vi "tutorial-062_FromDLAY.vi"(11 "Control Array":refnum<vi>[](array[refnum])) -> ()   [LabVIEW 2019]
uses:
  TextControlledInstrum/TextControlledInstrum.lvlib
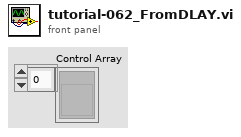
[diagram p1: front panel]
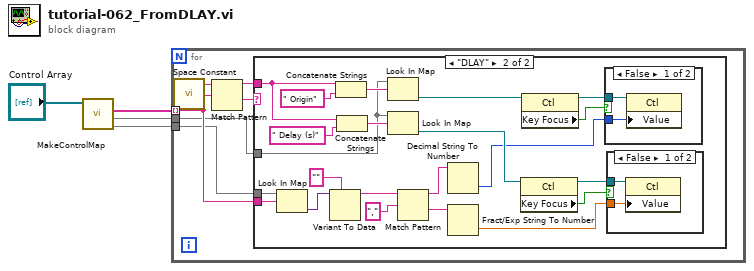
[diagram p0: block diagram]
diagram:
  n1 = call "MakeControlMap.vi"("ControlArray"="Control Array") -> ("ValueMap out"=w2:map{string, variant}, "ControlMap out"=w1:map{string, refnum<vi>}, "Names"=w3:string[])  [unwired: 7 in, 1 out]
  n2 = for {
    tunnel: w3 -> [w7] mode=indexing
    tunnel: w2 -> [w6]
    tunnel: w1 -> [w5]
    n3 = call <vilib>:"Space Constant.vi"() -> ("String"=w10:string)
    n4 = Match Pattern(string=w7, regular expression=w10) -> (before substring=w8:string, after substring=w9:string)  [unwired: 1 in, 2 out]
    n5 = case shown="\"DLAY\"" w9 {
      tunnel: w8 -> [_ w24]
      tunnel: w7 -> [_ w32]
      tunnel: w6 -> [_ w31]
      tunnel: w5 -> [_ w19]
      frame Default {
      }
      frame "DLAY" {
        n6 = Look In Map(map=w31, key=w32) -> (value=w25:variant)  [unwired: 1 in, 1 out]
        n7 = Variant To Data(type="", Variant=w25) -> (data=w26:string)  [unwired: 1 in, 1 out]
        n8 = Concatenate Strings(w24, " Origin") -> (w21:string)
        n9 = Concatenate Strings(w24, " Delay (s)") -> (w20:string)
        n10 = Look In Map(map=w19, key=w21) -> (value=w18:refnum<vi>)  [unwired: 1 in, 1 out]
        n11 = Look In Map(map=w19, key=w20) -> (value=w17:refnum<vi>)  [unwired: 1 in, 1 out]
        n12 = Match Pattern(string=w26, regular expression=",") -> (before substring=w27:string, after substring=w28:string)  [unwired: 1 in, 2 out]
        n13 = Decimal String To Number(string=w27) -> (number=w13:i32)  [unwired: 2 in, 1 out]
        n14 = Fract/Exp String To Number(string=w28) -> (number=w16:dbl)  [unwired: 3 in, 1 out]
        n15 = property class="Ctl"(reference=w17) -> (reference out=w14:refnum<vi>, "Key Focus"=w11:bool)  [unwired: 1 in, 1 out]
        n16 = property class="Ctl"(reference=w18) -> (reference out=w15:refnum<vi>, "Key Focus"=w12:bool)  [unwired: 1 in, 1 out]
        n17 = case shown="False" w12 {
          tunnel: w15 -> [w36 _]
          tunnel: w13 -> [w35 _]
          frame False {
            n18 = property class="Ctl"(reference=w36, "Value"=w35) -> ()  [unwired: 1 in, 2 out]
          }
          frame True {
          }
        }
        n19 = case shown="False" w11 {
          tunnel: w16 -> [w34 _]
          tunnel: w14 -> [w33 _]
          frame False {
            n20 = property class="Ctl"(reference=w33, "Value"=w34) -> ()  [unwired: 1 in, 2 out]
          }
          frame True {
          }
        }
      }
    }
  }
